vi "First Step.vi"(8 "error in (no error)":errorcluster, 11 "Magna Power Scan.lvclass in":refnum<class "Magna Power Scan.lvclass">) -> (0 "error out":errorcluster, 2 "Current Position":dbl, 3 "Magna Power Scan.lvclass out":refnum<class "Magna Power Scan.lvclass">)   [LabVIEW 2012, in "Magna Power Scan.lvclass"]
doc: "(Dynamic) Reset the instrument and prepare to scan. Go to step #0 - the first step. If desired, the scanner may do this in a different way than usual (i.e. by preparing to move a long distance, or reset to home position.)"
uses:
  Magna Power Scan.lvclass
  Instruments/Magna-Power Power Supply/Magna Power.lvclass
  Magna Power Scan.lvclass/Magna Power Scan.ctl
  Scanner/Scanner.lvclass
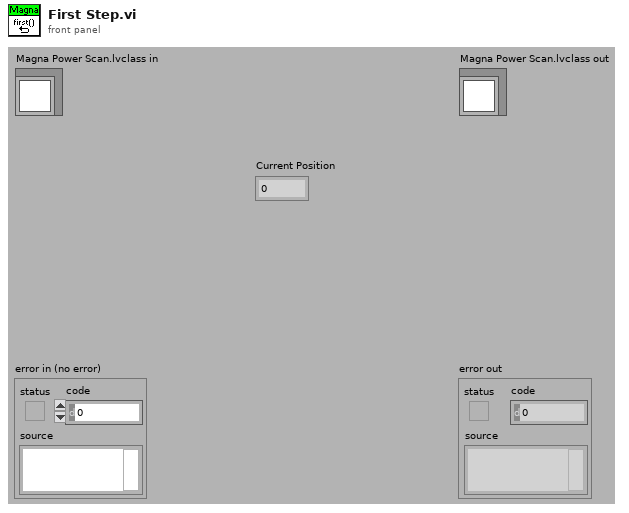
[diagram p1: front panel]
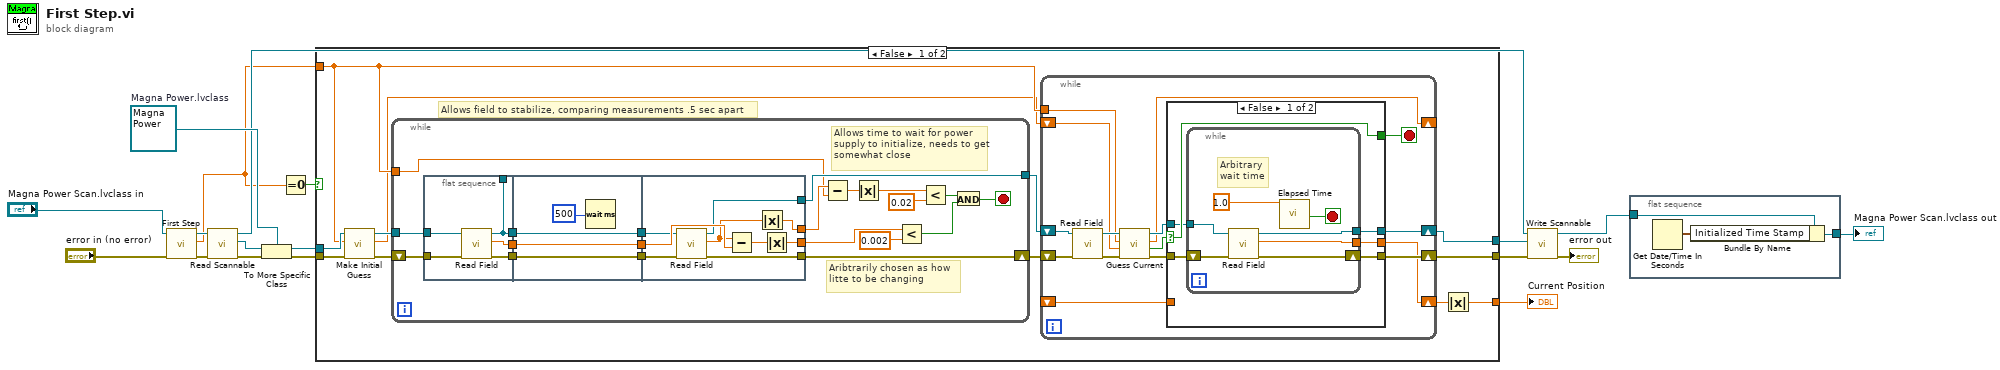
[diagram p0: block diagram]
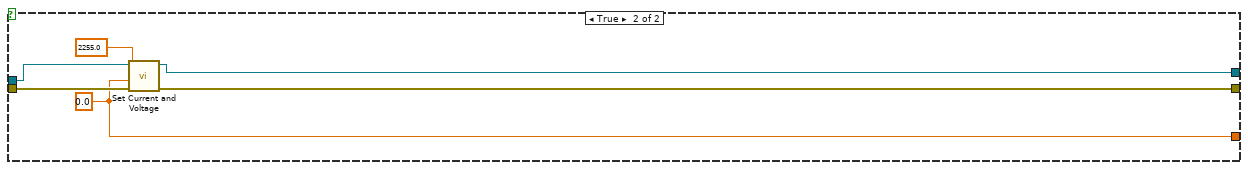
[diagram p3: hidden frame]
diagram:
  w14 = refnum<class "Magna Power.lvclass"> refnum  # Magna Power.lvclass
  n1 = call-parent "First Step.vi"("error in (no error)"="error in (no error)", "Scanner.lvclass in"="Magna Power Scan.lvclass in") -> ("error out"=w16:errorcluster, "Current Position"=w1:dbl, "Scanner.lvclass out"=w15:refnum<class "Magna Power Scan.lvclass">)  [unwired: 7 in]
  n2 = call-dynamic "Read Scannable.vi"("error in (no error)"=w16, "Scanner.lvclass in"=w15) -> ("error out"=w12:errorcluster, "Scannable.lvclass"=w13:refnum<class "Scannable.lvclass">, "Scanner.lvclass out"=w6:refnum<class "Magna Power Scan.lvclass">)  [unwired: 7 in]
  n3 = To More Specific Class(target class=w14, reference=w13, error in=w12) -> (specific class reference=w10:refnum<class "Magna Power.lvclass">, error out=w11:errorcluster)
  n4 = Equal To 0?(x=w1) -> (x = 0?=w2:bool)
  n5 = case shown="False" w2 {
    tunnel: w11 -> [w26 w106]
    tunnel: w10 -> [w25 w105]
    tunnel: w1 -> [w24 _]
    tunnel: [w19 w102] -> w9
    tunnel: [w22 w103] -> w8
    tunnel: [w21 w101] -> w7
    frame False {
      # "Allows field to stabilize, comparing measurements .5 sec apart"
      n6 = call "Make Initial Guess.vi"("error in (no error)"=w26, "Desired Field"=w24, "Magna Power in"=w25) -> ("error out"=w27:errorcluster, "First guess"=w23:dbl, "Magna Power out"=w28:refnum<class "Magna Power.lvclass">)  [unwired: 6 in]
      n7 = while {
        shift-right: [w76] -> w30
        shift-left: w27 -> [w82]
        tunnel: w28 -> [w74]
        tunnel: [w71] -> w29
        tunnel: w24 -> [w67]
        stop <- w70 stop-if-true
        # "Aribtrarily chosen as how litte to be changing"
        # "Allows time to wait for power supply to initialize, needs to get somewhat close"
        n8 = flat-sequence {
          tunnel: w82 -> [w87]
          tunnel: [w86] -> w80
          tunnel: [w85] -> w78
          tunnel: w74 -> [w84]
          tunnel: [w83] -> w72
          tunnel: [w83] -> _
          tunnel: [w90] -> w81
          tunnel: w80 -> [w90]
          tunnel: [w89] -> w79
          tunnel: w78 -> [w89]
          tunnel: [w88] -> w73
          tunnel: w72 -> [w88]
          tunnel: w81 -> [w100]
          tunnel: w79 -> [w98]
          tunnel: [w97] -> w75
          tunnel: [w96] -> w76
          tunnel: w73 -> [w94]
          tunnel: [w95] -> w71
          tunnel: [w92] -> w68
          frame #0 {
            n9 = call "Read Field.vi"("error in (no error)"=w87, "Magna Power in"=w84) -> ("error out"=w86:errorcluster, "Field (T)"=w85:dbl, "Magna Power out"=w83:refnum<class "Magna Power.lvclass">)  [unwired: 7 in]
          }
          frame #1 {
            n10 = Wait (ms)(milliseconds to wait=u32 500) -> ()  [unwired: 1 out]
          }
          frame #2 {
            n11 = call "Read Field.vi"("error in (no error)"=w100, "Magna Power in"=w94) -> ("error out"=w96:errorcluster, "Field (T)"=w93:dbl, "Magna Power out"=w95:refnum<class "Magna Power.lvclass">)  [unwired: 7 in]
            n12 = Subtract(x=w93, y=w98) -> (x-y=w99:dbl)
            n13 = Absolute Value(x=w93) -> (abs(x)=w92:dbl)
            n14 = Absolute Value(x=w99) -> (abs(x)=w97:dbl)
          }
        }
        n15 = Subtract(x=w68, y=w67) -> (x-y=w66:dbl)
        n16 = Absolute Value(x=w66) -> (abs(x)=w65:dbl)
        n17 = Less?(x=w75, y=0.002) -> (x < y?=w69:bool)
        n18 = Less?(x=w65, y=0.02) -> (x < y?=w63:bool)
        n19 = And(x=w63, y=w69) -> (x .and. y?=w70:bool)
      }
      n20 = while {
        shift-right: [w41] -> w22
        shift-left: w30 -> [w45]
        shift-right: [w36] -> w21
        shift-left: w29 -> [w40]
        tunnel: w24 -> [w35]
        shift-right: [w32] -> _
        shift-left: w23 -> [w33]
        shift-right: [w34] -> w20
        shift-left: _ -> [w31]
        stop <- w38 stop-if-true
        n21 = call "Read Field.vi"("error in (no error)"=w45, "Magna Power in"=w40) -> ("error out"=w44:errorcluster, "Magna Power out"=w37:refnum<class "Magna Power.lvclass">)  [unwired: 7 in, 1 out]
        n22 = call "Guess Current.vi"("error in (no error)"=w44, "Current guess"=w33, "Desired Field"=w35, "Magna Power in"=w37) -> ("error out"=w42:errorcluster, "Stop?"=w43:bool, "New guess"=w32:dbl, "Magna Power out"=w39:refnum<class "Magna Power.lvclass">)  [unwired: 4 in]
        n23 = case shown="False" w43 {
          selector: w43 -> [w50 w62]
          tunnel: [w50 w62] -> w38
          tunnel: w42 -> [w51 w61]
          tunnel: [w49 w61] -> w41
          tunnel: w39 -> [w48 w60]
          tunnel: [w47 w60] -> w36
          tunnel: [w46 w59] -> w34
          tunnel: w31 -> [_ w59]
          frame False {
            n24 = while {
              shift-right: [w57] -> w49
              shift-left: w51 -> [w58]
              tunnel: w48 -> [w55]
              tunnel: [w53] -> w47
              tunnel: [w52] -> w46
              stop <- w54 stop-if-true
              # "Arbitrary\nwait time"
              n25 = call "Read Field.vi"("error in (no error)"=w58, "Magna Power in"=w55) -> ("error out"=w57:errorcluster, "Field (T)"=w52:dbl, "Magna Power out"=w53:refnum<class "Magna Power.lvclass">)  [unwired: 7 in]
              n26 = call "Elapsed Time"("Time Target (s)"=1.0) -> ("Time has Elapsed"=w54:bool)  [unwired: 11 in, 7 out]
            }
          }
          frame True {
          }
        }
      }
      n27 = Absolute Value(x=w20) -> (abs(x)=w19:dbl)
    }
    frame True {
      w102 = 0.0 ("Current Limit")
      n28 = call "Set Current and Voltage.vi"("error in (no error)"=w106, "Current Limit"=w102, "Voltage Limit"=2255.0, "Magna Power in"=w105) -> ("error out"=w103:errorcluster, "Magna Power out"=w101:refnum<class "Magna Power.lvclass">)  [unwired: 6 in]
    }
  }
  "Current Position" <- w9
  n29 = call-dynamic "Write Scannable.vi"("error in (no error)"=w8, "Scannable.lvclass"=w7, "Scanner.lvclass in"=w6) -> ("error out"=→"error out":errorcluster, "Scanner.lvclass out"=w4:refnum<class "Magna Power Scan.lvclass">)  [unwired: 7 in]
  n30 = flat-sequence {
    tunnel: w4 -> [w108]
    tunnel: [w107] -> w3
    frame #0 {
      n31 = Get Date/Time In Seconds() -> (seconds since 1Jan1904=w109:timestamp)
      n32 = Bundle By Name(cluster=w108, "Initialized Time Stamp"=w109) -> (w107:refnum<class "Magna Power Scan.lvclass">)
    }
  }
  "Magna Power Scan.lvclass out" <- w3
